vi "ReadMerecuryITC.vi"() -> ()   [LabVIEW 2014]
panel:
  in  "error in (no error)":errorcluster
  out "error out":errorcluster
  out "String 4":string
  in  "String":string
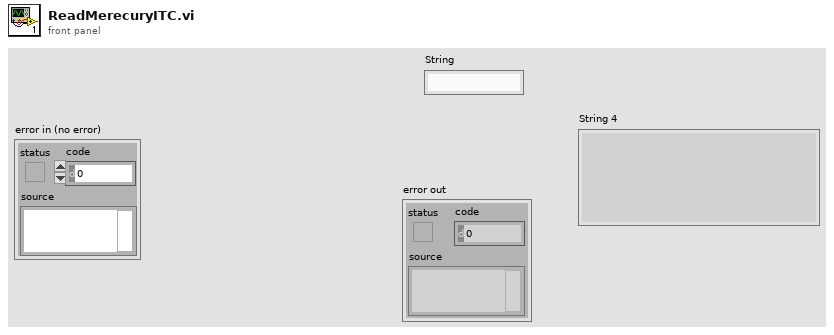
[diagram p1: front panel]
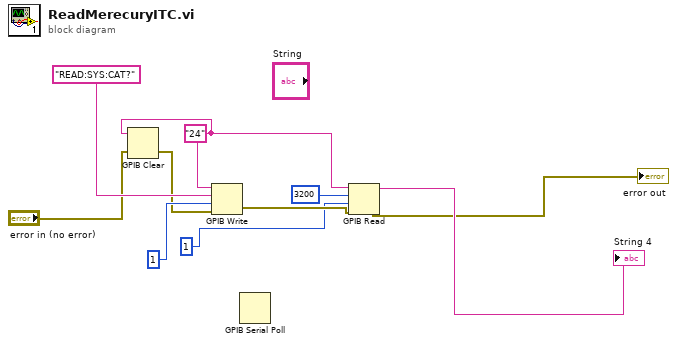
[diagram p0: block diagram]
diagram:
  w3 = "24"
  n1 = GPIB Clear(2:"error in (no error)", 3:w3) -> (0:w1:errorcluster)  [unwired: 1 out]
  n2 = GPIB Write(0:w3, 1:"READ:SYS:CAT?", 2:1, 3:w1) -> (6:w10:errorcluster)  [unwired: 1 in, 1 out]
  n3 = GPIB Serial Poll() -> ()  [unwired: 2 in, 3 out]
  n4 = GPIB Read(0:w3, 1:3200, 2:1, 3:w10) -> (5:→"String 4":string, 7:→"error out":errorcluster)  [unwired: 1 in, 1 out]
